vi "Pockels Cal-Set graph plot legend.vi"(8 "error in (no error)":errorcluster, 10 "Cal data header":string[](array[string]), 11 "XYGraph in":refnum<vi>) -> (0 "error out":errorcluster, 2 "Number of cal curves":i32, 3 "XYGraph out":refnum<vi>)   [LabVIEW 2013]
uses:
  Globals/gl_Calibration globals.vi
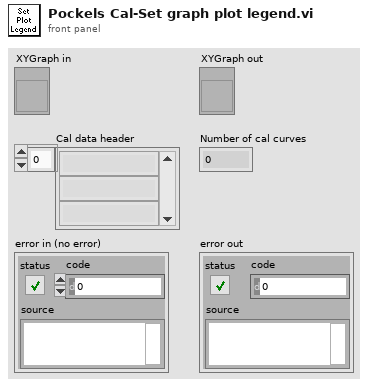
[diagram p1: front panel]
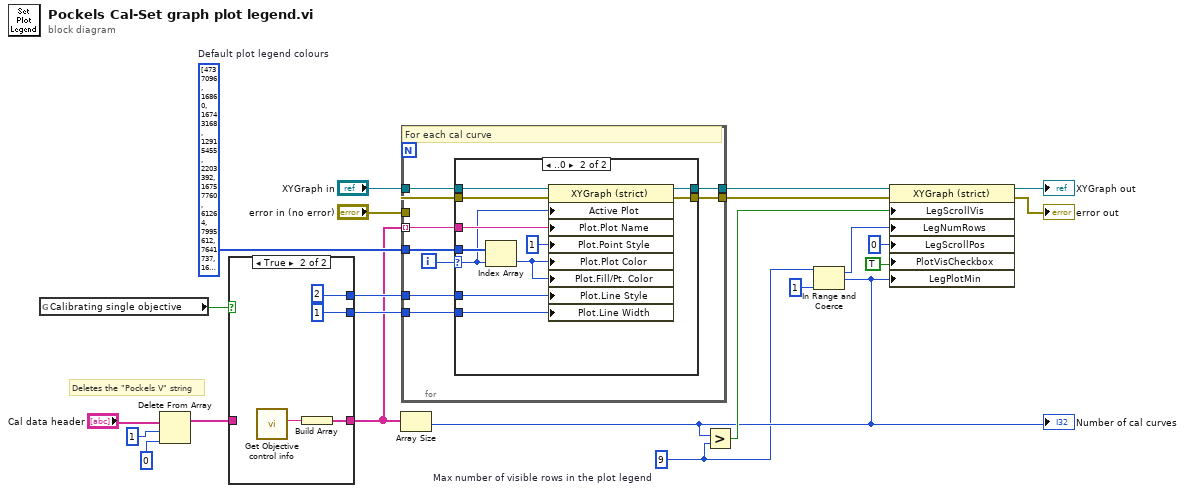
[diagram p0: block diagram]
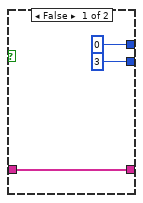
[diagram p2: hidden frame]
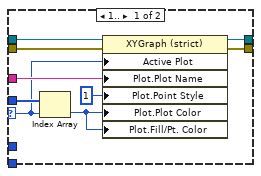
[diagram p3: hidden frame]
diagram:
  w6 = u32[] [4737096, 16860, 16743168, 12915455, 2203392, 16757760, 61264, 7995612, 7641737, 16750610, 9934743, 10420301]  # Default plot legend colours
  w7 = 9  # Max number of visible rows in the plot legend
  # "Deletes the \"Pockels V\" string"
  n1 = global read "gl_Calibration globals.vi" "Calibrating single objective"() -> (w5:bool)
  n2 = Delete From Array "Delete From Array"(array="Cal data header", length=1, index=0) -> (array with subset deleted=w2:string[])  [unwired: 1 out]
  n3 = case shown="True" w5 {
    tunnel: [u8 0 u8 2] -> w4
    tunnel: [u8 3 ("Plot.Line Width") u8 1 ("Plot.Line Width")] -> w3
    tunnel: w2 -> [w23 _]
    tunnel: [w23 w27] -> w1
    frame False {
    }
    frame True {
      n4 = call "Get Objective control info.vi"() -> ("Value"=w26:string)  [unwired: 7 in, 4 out]
      n5 = Build Array(w26) -> (w27:string[])
    }
  }
  n6 = Array Size(array=w1) -> (size(s)=w8:i32)
  "Number of cal curves" <- w8
  n7 = for {
    tunnel: "XYGraph in" -> [w35]
    tunnel: "error in (no error)" -> [w34]
    tunnel: [w38] -> w15
    tunnel: [w37] -> w14
    tunnel: w1 -> [w36] mode=indexing
    tunnel: w6 -> [w33]
    tunnel: w4 -> [w31]
    tunnel: w3 -> [w30]
    i -> [w32]
    # "For each cal curve"
    n8 = case shown="..0" w32 {
      selector: w32 -> [w39 w50]
      tunnel: [w47 w58] -> w38
      tunnel: [w46 w57] -> w37
      tunnel: w36 -> [w45 w56]
      tunnel: w35 -> [w44 w55]
      tunnel: w34 -> [w43 w54]
      tunnel: w33 -> [w41 w52]
      tunnel: w31 -> [_ w49]
      tunnel: w30 -> [_ w48]
      frame 1.. {
        n9 = Index Array(array=w41, index=w39) -> (element=w40:u32)
        n10 = property on="Property Node" class="XYGraph (strict)"(reference=w44, error in=w43, "Active Plot"=w39, "Plot.Plot Name"=w45, "Plot.Point Style"=u8 1 ("Plot.Bar Plot Style"), "Plot.Plot Color"=w40, "Plot.Fill/Pt. Color"=w40) -> (reference out=w46:refnum<vi>, error out=w47:errorcluster)
      }
      frame ..0 {
        n11 = Index Array(array=w52, index=w50) -> (element=w51:u32)
        n12 = property on="Property Node" class="XYGraph (strict)"(reference=w55, error in=w54, "Active Plot"=w50, "Plot.Plot Name"=w56, "Plot.Point Style"=u8 1 ("Plot.Bar Plot Style"), "Plot.Plot Color"=w51, "Plot.Fill/Pt. Color"=w51, "Plot.Line Style"=w49, "Plot.Line Width"=w48) -> (reference out=w57:refnum<vi>, error out=w58:errorcluster)
      }
    }
  }
  n13 = Greater?(x=w8, y=w7) -> (0:w13:bool)
  n14 = In Range and Coerce(upper limit=w7, x=w8, lower limit=1) -> (coerced(x)=w12:i32)  [unwired: 1 out]
  n15 = property on="Property Node" class="XYGraph (strict)"(reference=w14, error in=w15, "LegScrollVis"=w13, "LegNumRows"=w12, "LegScrollPos"=u32 0 ("Legend:Scroll Position"), "PlotVisCheckbox"=TRUE ("Legend:Plot Visibility Checkbox Visible"), "LegPlotMin"=w8) -> (reference out=→"XYGraph out":refnum<vi>, error out=→"error out":errorcluster)
